vi "Dequeue Message With Timeout.vi"(8 "error in (no error)":errorcluster, 9 "Timeout in ms (-1)":i32, 11 "Queue In":refnum<queue>) -> (0 "error out":errorcluster, 1 "Message Data":variant, 2 "Message":string, 3 "Queue Out":refnum<queue>, 4 "timed out?":bool)   [LabVIEW 2014, in "Message Queue.lvlib"]
uses:
  Message Queue.lvlib
  Message Cluster.ctl
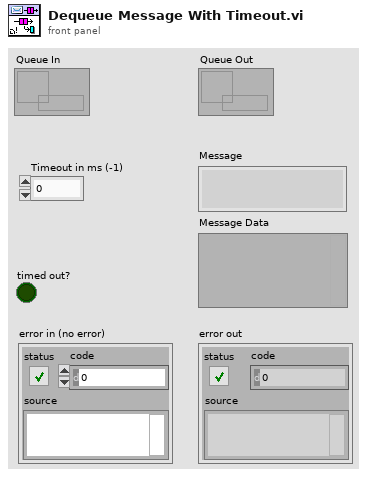
[diagram p1: front panel]
types:
  T1 = typedef "Message Queue.lvlib/Message Cluster.ctl" = cluster{"Message":string, "Message Data":variant}
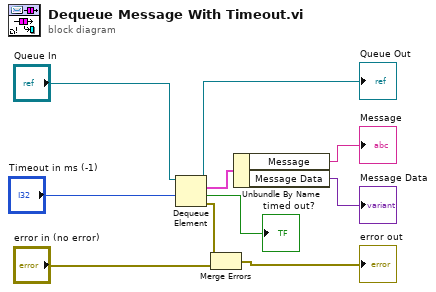
[diagram p0: block diagram]
diagram:
  n1 = Dequeue Element(queue="Queue In", timeout in ms (-1)="Timeout in ms (-1)") -> (queue out=→"Queue Out":refnum<queue>, element=w6:T1, timed out?=→"timed out?":bool, error out=w8:errorcluster)  [unwired: 1 in]
  n2 = Merge Errors(w8, "error in (no error)") -> (→"error out":errorcluster)
  n3 = Unbundle By Name(w6) -> ("Message"=→"Message":string, "Message Data"=→"Message Data":variant)
